vi "Ramp_Integrator.vi"(1 "tsample":sgl, 2 "w":sgl) -> (0 "theta":sgl)   [LabVIEW 2013]
panel:
  # "This VI is configured as Non-reentrant. \nOnly ONE copy of the Vi actually exists on the FPGA hardware."
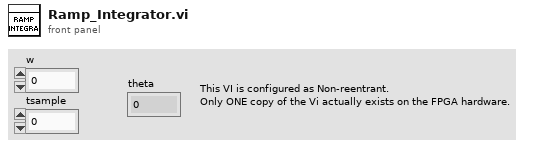
[diagram p1: front panel]
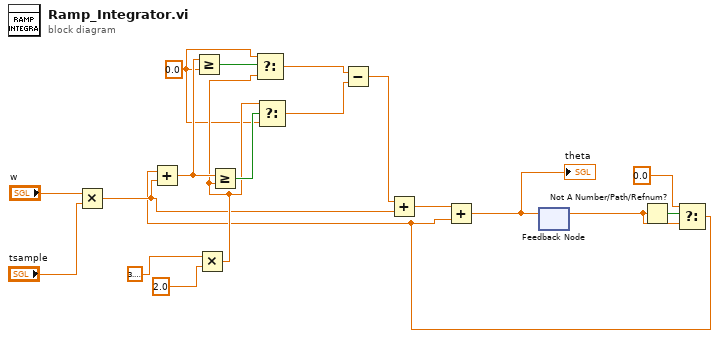
[diagram p0: block diagram]
diagram:
  w12 = sgl 0.0 ("y")
  n1 = Multiply(x="w", y="tsample") -> (x*y=w8:sgl)
  n2 = Multiply(x=sgl 3.1415927, y=sgl 2.0) -> (x*y=w13:sgl)
  n3 = feedback #1() -> (w2:sgl)  [unwired: 1 in]
  n4 = Not A Number/Path/Refnum?(number/path/refnum=w2) -> (NaN/Path/Refnum?=w5:bool)
  n5 = Select(t=sgl 0.0, s=w5, f=w2) -> (s? t:f=w1:sgl)
  n6 = Add(x=w1, y=w8) -> (x+y=w15:sgl)
  n7 = Greater Or Equal?(x=w15, y=w12) -> (x >= y?=w16:bool)
  n8 = Greater Or Equal?(x=w15, y=w13) -> (x >= y?=w17:bool)
  n9 = Select(t=w12, s=w16, f=w13) -> (s? t:f=w11:sgl)
  n10 = Select(t=w13, s=w17, f=w12) -> (s? t:f=w10:sgl)
  n11 = Subtract(x=w11, y=w10) -> (x-y=w9:sgl)
  n12 = Add(x=w9, y=w8) -> (x+y=w7:sgl)
  n13 = Add(x=w7, y=w1) -> (x+y=w3:sgl)
  "theta" <- w3
  n14 = feedback-in #1(w3) -> ()
